vi "TEMPDo.vi"(8 "error in (no error)":errorcluster, 10 "Actor in":refnum<class "Actor.lvclass">, 11 "DNL_Message Template":refnum<class "Message.lvclass">) -> (0 "error out":errorcluster, 2 "Actor out":refnum<class "Actor.lvclass">)   [LabVIEW 2015, in "Dialog PV Template.lvclass"]
doc: "This VI delivers the message to the actor by calling the appropriate method(s) on the actor."
uses:
  Dialog PV Template.lvclass
  <vilib>/ActorFramework/Actor/Actor.lvclass
  <vilib>/ActorFramework/Message/Message.lvclass
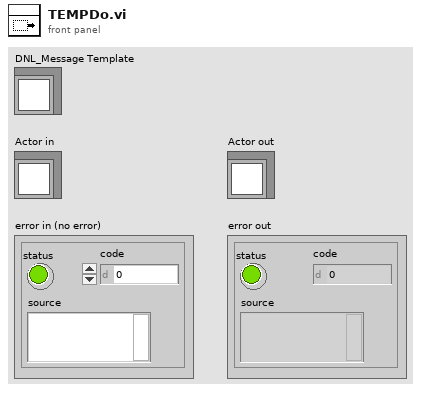
[diagram p1: front panel]
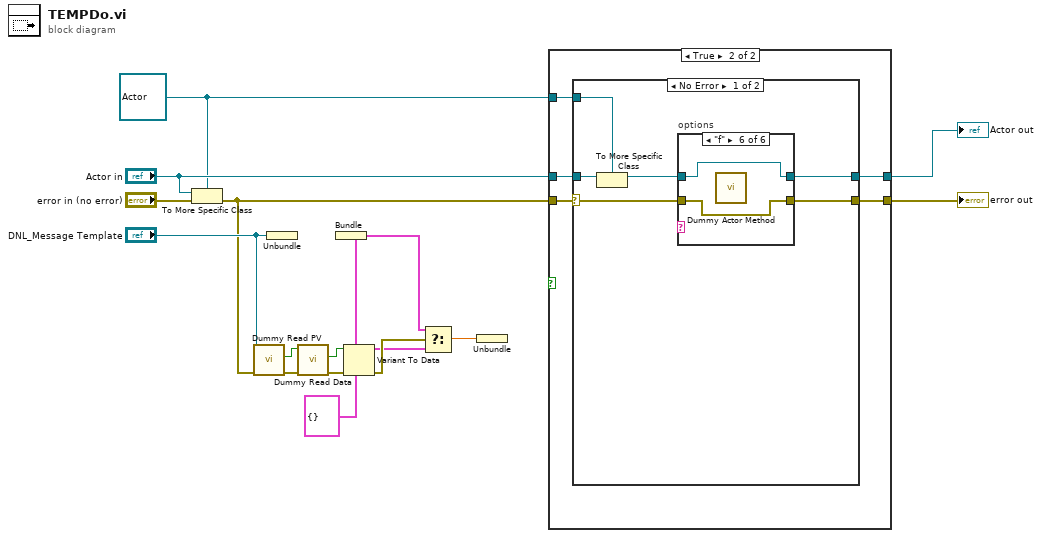
[diagram p0: block diagram]
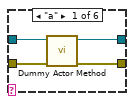
[diagram p3: hidden frame]
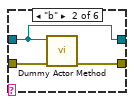
[diagram p4: hidden frame]
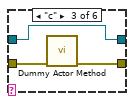
[diagram p5: hidden frame]
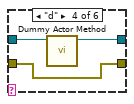
[diagram p6: hidden frame]
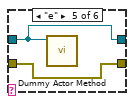
[diagram p7: hidden frame]
diagram:
  w2 = cluster{} {} ("Type")
  w12 = refnum<class "Actor.lvclass"> refnum ("Actor in")
  n1 = To More Specific Class(target class=w12, reference="Actor in", error in="error in (no error)") -> (error out=w10:errorcluster)  [unwired: 1 out]
  n2 = call "Dummy Read PV.vi"("error in (no error)"=w10, "Actor in"="DNL_Message Template") -> ("error out"=w9:errorcluster, "Boolean"=w1:bool)  [unwired: 7 in, 1 out]
  n3 = Unbundle ("Pre-Unbundler")("DNL_Message Template") -> ()  [unwired: 1 out]
  n4 = call "Dummy Read Data.vi"("error in (no error)"=w9, "Actor in"=w1) -> ("error out"=w7:errorcluster, "Boolean"=w8:bool)  [unwired: 7 in, 1 out]
  n5 = Bundle ("Pre-Bundler")(cluster=w2) -> (w5:cluster{void})  [unwired: 1 in]
  n6 = Variant To Data(error in=w7, type=w2, Variant=w8) -> (data=w4:cluster{}, error out=w6:errorcluster)
  n7 = Select(t=w5, s=w6, f=w4) -> (s? t:f=w3:dbl)
  n8 = Unbundle ("Main-Unbundler")(w3) -> ()  [unwired: 1 out]
  n9 = case "Execute?" shown="True" {
    selector: _ -> [_ _]
    tunnel: [w17 w23] -> w15
    tunnel: [w18 w22] -> w14
    tunnel: "Actor in" -> [w18 w21]
    tunnel: w12 -> [_ w20]
    tunnel: w10 -> [w17 w19]
    frame False {
    }
    frame True {
      n10 = case shown="No Error" w19 {
        selector: w19 -> [w27 w48]
        tunnel: [w29 w48] -> w23
        tunnel: [w28 w47] -> w22
        tunnel: w21 -> [w26 w47]
        tunnel: w20 -> [w25 _]
        frame No Error {
          n11 = To More Specific Class(target class=w25, reference=w26) -> (specific class reference=w24:refnum<class "Actor.lvclass">)  [unwired: 1 in, 1 out]
          n12 = case "options" shown="\"f\"" {
            selector: _ -> [_ _ _ _ _ _]
            tunnel: [w33 w36 w39 w42 w43 w45] -> w29
            tunnel: [w32 w34 w37 w40 w44 w46] -> w28
            tunnel: w27 -> [w31 w35 w38 w42 w43 w45]
            tunnel: w24 -> [w30 w34 w37 w41 w44 w46]
            frame "a" {
              n13 = call "Dummy Actor Method.vi"("error in (no error)"=w31, "Actor in"=w30) -> ("error out"=w33:errorcluster, "Actor out"=w32:refnum<class "Actor.lvclass">)  [unwired: 8 in]
            }
            frame "b" {
              n14 = call "Dummy Actor Method.vi"("error in (no error)"=w35, "Actor in"=w34) -> ("error out"=w36:errorcluster)  [unwired: 8 in, 1 out]
            }
            frame "c" {
              n15 = call "Dummy Actor Method.vi"("error in (no error)"=w38) -> ("error out"=w39:errorcluster)  [unwired: 9 in, 1 out]
            }
            frame "d" {
              n16 = call "Dummy Actor Method.vi"("Actor in"=w41) -> ("Actor out"=w40:refnum<class "Actor.lvclass">)  [unwired: 9 in, 1 out]
            }
            frame "e" {
              n17 = call "Dummy Actor Method.vi"("Actor in"=w44) -> ()  [unwired: 9 in, 2 out]
            }
            frame "f" {
              n18 = call "Dummy Actor Method.vi"() -> ()  [unwired: 10 in, 2 out]
            }
          }
        }
        frame Error {
        }
      }
    }
  }
  "error out" <- w15
  "Actor out" <- w14
